vi "Main.vi"   [LabVIEW 2018]
uses:
  Architecture/Modules.ctl
types:
  T1 = typedef "Modules.ctl" = enum16{"Database", "Car Wash Controller", "Console"}
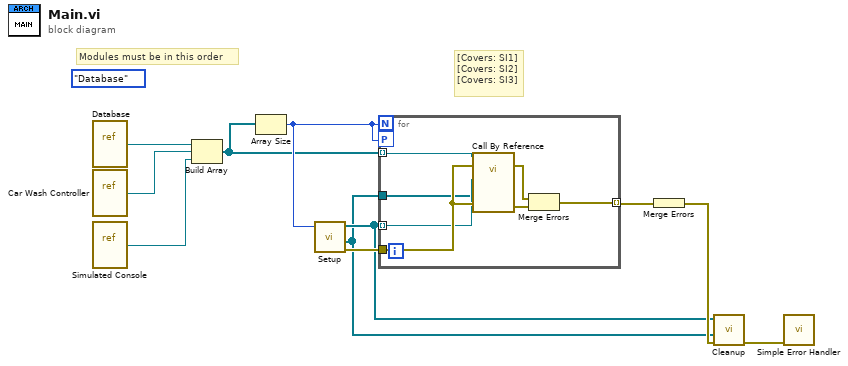
[diagram p0: block diagram]
diagram:
  (unwired) Modules."Database" ("Modules")
  # "[Covers: SI1]\n[Covers: SI2]\n[Covers: SI3]"
  # "Modules must be in this order"
  n1 = vi-ref "Database.vi"() -> (w2:refnum<vi>)
  n2 = vi-ref "Car Wash Controller.vi"() -> (w11:refnum<vi>)
  n3 = vi-ref "Simulated Console.vi"() -> (w3:refnum<vi>)
  n4 = Build Array(w2, w11, w3) -> (w9:refnum<vi>[])
  n5 = Array Size(array=w9) -> (size(s)=w10:i32)
  n6 = call "Setup.vi"("Number of Modules"=w10) -> ("error out"=w8:errorcluster, "Module Routes"=w4:refnum<user-event>[], "Event Refs"=w5:refnum<event-registration>[])  [unwired: 8 in]
  n7 = for {
    N: w10 -> [_]
    workers-P: w10 -> [_]
    tunnel: w9 -> [w18] mode=indexing
    tunnel: w8 -> [w17]
    tunnel: w5 -> [w16] mode=indexing
    tunnel: w4 -> [w15]
    tunnel: [w12] -> w7 mode=indexing
    n8 = call-by-ref "?"(reference=w18, error in=w17, 8:"error in (no error)"=w17, "Module Routes"=w15, "Event Registration Refnum"=w16) -> (error out=w13:errorcluster, 0:"error out"=w14:errorcluster)  [unwired: 8 in, 1 out]
    n9 = Merge Errors(w13, w14) -> (w12:errorcluster)
  }
  n10 = Merge Errors(w7) -> (w6:errorcluster)
  n11 = call "Cleanup.vi"("error in (no error)"=w6, "Module Routes"=w4, "Event Refs"=w5) -> ("error out"=w1:errorcluster)  [unwired: 8 in]
  n12 = call <vilib>:"Simple Error Handler.vi"("error in (no error)"=w1) -> ()  [unwired: 4 in, 5 out]
